vi "CSV Row Selector.vi"(4 "Time Column Index":i32, 6 "delimiter (,)":string=",", 10 "file path (dialog if empty)":path=path "C:/Users/Marvi/Desktop/code/sandbox/ni/csv_row_selection_tool/config/motor_schedule.csv", 11 "Current Time (msec)":i64) -> (0 "All Rows":string[][](array[string]), 2 "Elapsed Time":dbl, 3 "Selected Rows":string[][](array[string]))   [LabVIEW 2020]
uses:
  <vilib>/Utility/file.llb/Read Delimited Spreadsheet (string).vi
panel:
  out "element":i32
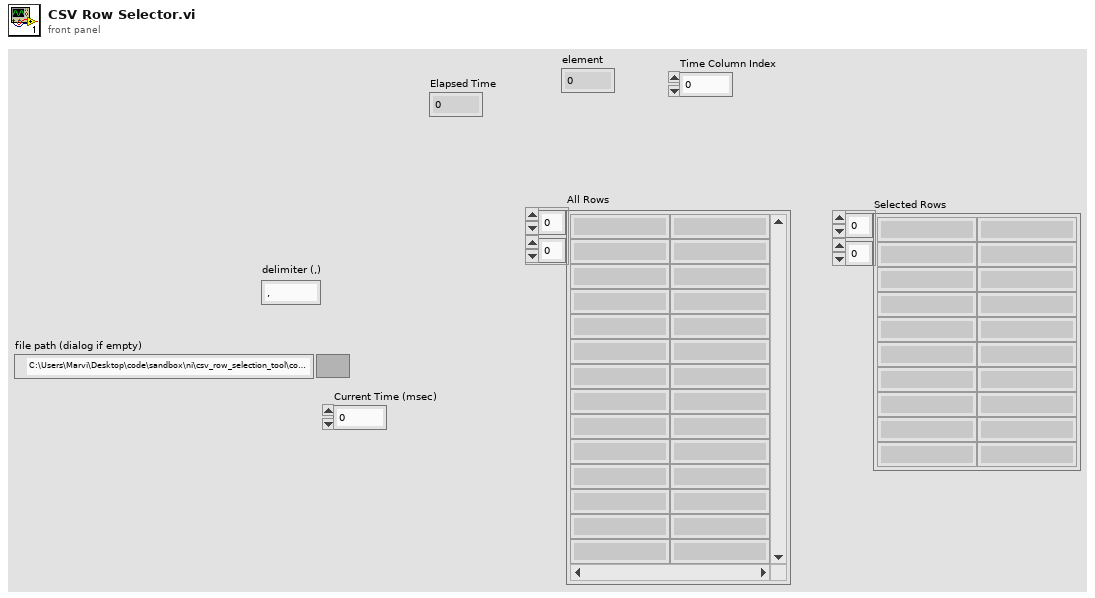
[diagram p1: front panel]
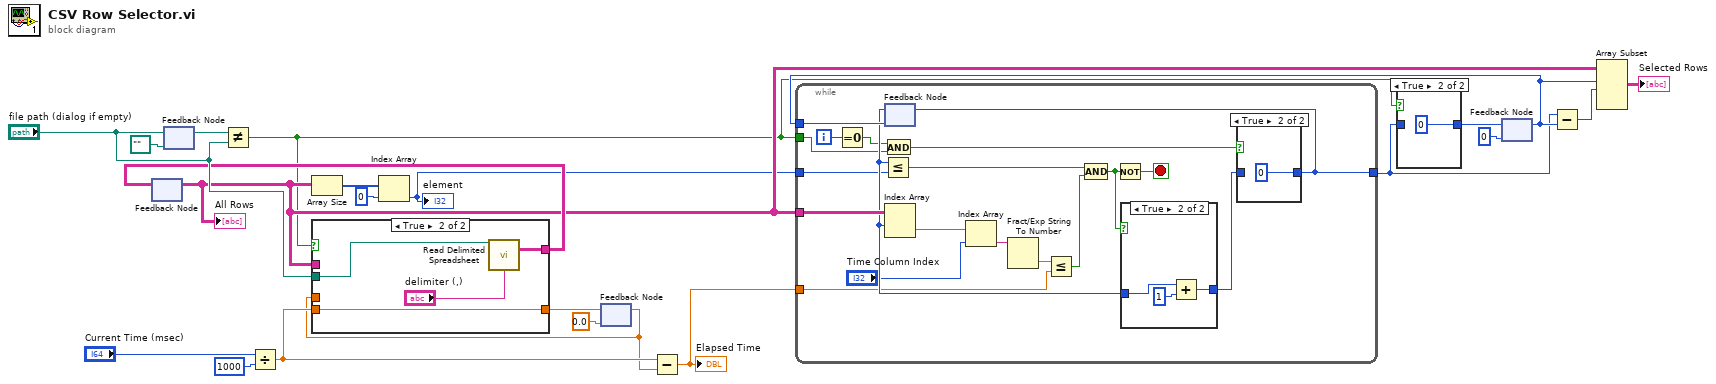
[diagram p0: block diagram]
diagram:
  n1 = feedback #1() -> (w7:string[][])  [unwired: 1 in]
  "All Rows" <- w7
  n2 = feedback-in #2("file path (dialog if empty)") -> ()
  n3 = feedback #2(path "" ("file path (dialog if empty)")) -> (w21:path)
  n4 = Not Equal?(x=w21, y="file path (dialog if empty)") -> (x != y?=w1:bool)
  n5 = Divide(x="Current Time (msec)", y=i64 1000 ("x")) -> (x/y=w15:dbl)
  n6 = Array Size(array=w7) -> (size(s)=w13:i32[])
  n7 = Index Array(array=w13, index=0) -> (element=w4:i32)
  "element" <- w4
  n8 = feedback #3(0.0) -> (w14:dbl)
  n9 = case shown="True" w1 {
    tunnel: [w24 w26] -> w11
    tunnel: "file path (dialog if empty)" -> [_ w28]
    tunnel: w7 -> [w24 _]
    tunnel: [w23 w25] -> w17
    tunnel: w15 -> [_ w25]
    tunnel: w14 -> [w23 _]
    frame False {
    }
    frame True {
      n10 = call-poly <vilib>:"Read Delimited Spreadsheet.vi"("file path (dialog if empty)"=w28, "delimiter (\\t)"="delimiter (,)") -> ("all rows"=w26:string[][])  [unwired: 8 in, 5 out]
    }
  }
  n11 = feedback-in #1(w11) -> ()
  n12 = feedback-in #3(w17) -> ()
  n13 = Subtract(x=w15, y=w14) -> (x-y=w6:dbl)
  "Elapsed Time" <- w6
  n14 = feedback #4(0) -> (w5:i32)
  n15 = while {
    tunnel: [w34] -> w3
    tunnel: w7 -> [w47]
    tunnel: w5 -> [w44]
    tunnel: w4 -> [w39]
    tunnel: w6 -> [w37]
    tunnel: w1 -> [w30]
    i -> [w32]
    stop <- w45 stop-if-true
    n16 = Equal To 0?(x=w32) -> (x = 0?=w29:bool)
    n17 = And(x=w29, y=w30) -> (x .and. y?=w31:bool)
    n18 = feedback #5(w44) -> (w41:i32)
    n19 = Less Or Equal?(x=w41, y=w39) -> (x <= y?=w40:bool)
    n20 = Index Array(array=w47, index (row)=w41) -> (element=w46:string[])  [unwired: 1 in]
    n21 = Index Array(array=w46, index="Time Column Index") -> (element=w35:string)
    n22 = Fract/Exp String To Number(string=w35) -> (number=w36:dbl)  [unwired: 3 in, 1 out]
    n23 = Less Or Equal?(x=w36, y=w37) -> (x <= y?=w42:bool)
    n24 = Compound Arithmetic op=AND(w40, w42) -> (w43:bool)
    n25 = Not(x=w43) -> (.not. x?=w45:bool)
    n26 = case shown="True" w43 {
      tunnel: [w50 w52] -> w33
      tunnel: w41 -> [w50 w51]
      frame False {
      }
      frame True {
        n27 = Add(x=w51, y=1) -> (x+y=w52:i32)
      }
    }
    n28 = case shown="True" w31 {
      tunnel: [w48 0] -> w34
      tunnel: w33 -> [w48 _]
      frame False {
      }
      frame True {
      }
    }
    n29 = feedback-in #5(w34) -> ()
  }
  n30 = case shown="True" w1 {
    tunnel: w3 -> [w54 _]
    tunnel: [w54 0] -> w2
    frame False {
    }
    frame True {
    }
  }
  n31 = feedback-in #4(w2) -> ()
  n32 = Subtract(x=w3, y=w5) -> (x-y=w9:i32)
  n33 = Array Subset(array=w7, index (row)=w5, length (row)=w9) -> (→"Selected Rows":string[][])  [unwired: 2 in]
